vi "Binary (Approximate) Search 1D Array (DBL).vi"(1 "epsilon (machine)":dbl=2.220446049250313e-16, 2 "element":dbl format="%.2f", 3 "1D array":dbl[](array[numeric]) format="%.2f") -> (0 "index":i32)   [LabVIEW 2019]
doc: "This is a binary search through a 1D array. It has no start index input and searches the entire array for the element requested.\n\nIf found, the index of the match is returned. If not found, an index of -1 is returned.\n\nDue to the nature of the binary search, your input array must already be sorted. This function will not sort your array, so if you send in an unsorted array, it will not function properly. Furthermore, if you have duplicate elements in your array, it is not guaranteed that the index returned will be to the match with the lowest array element number.\n\nThis is the double-precision floating-point (DBL) portion of the polymorphic VI."
panel:
  # "Select Help»Show Context Help and move the cursor \nover the VI icon to display help for this VI."
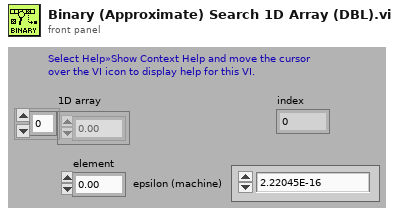
[diagram p1: front panel]
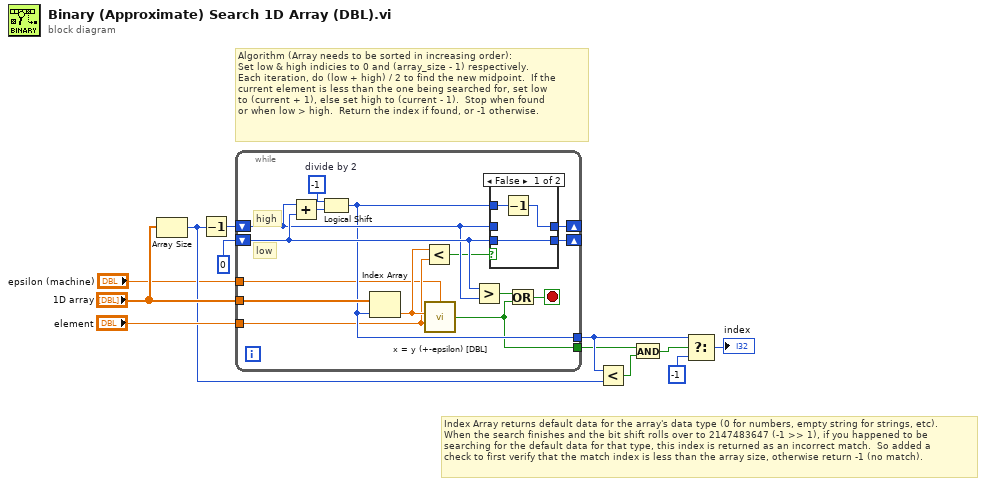
[diagram p0: block diagram]
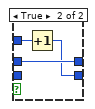
[diagram p2: hidden frame]
diagram:
  # "Index Array returns default data for the array's data type (0 for numbers, empty string for strings, etc).\nWhen the search finishes and the bit shift rolls over to 2147483647 (-1 >> 1), if you happened to be\nsearching for the default data for that type, this index is returned as an incorrect match.  So added a\ncheck to first verify that the match index is less than the array size, otherwise return -1 (no match)."
  # "Algorithm (Array needs to be sorted in increasing order):\nSet low & high indicies to 0 and (array_size - 1) respectively.\nEach iteration, do (low + high) / 2 to find the new midpoint.  If the\ncurrent element is less than the one being searched for, set low\nto (current + 1), else set high to (current - 1).  Stop when found\nor when low > high.  Return the index if found, or -1 otherwise."
  n1 = Array Size(array="1D array") -> (size(s)=w2:i32)
  n2 = Decrement(x=w2) -> (x-1=w9:i32)
  n3 = while {
    tunnel: "1D array" -> [w27]
    tunnel: "element" -> [w14]
    shift-right: [w23] -> _
    shift-left: w9 -> [w20]
    tunnel: [w16] -> w4
    shift-right: [w22] -> _
    shift-left: 0 -> [w21]
    tunnel: [w18] -> w5
    tunnel: "epsilon (machine)" -> [w13]
    stop <- w26 stop-if-true
    w24 = -1  # divide by 2
    # "low"
    # "high"
    n4 = Add(x=w20, y=w21) -> (x+y=w25:i32)
    n5 = Logical Shift(y=w24, x=w25) -> (x << y=w18:i32)
    n6 = Index Array(array=w27, index=w18) -> (element=w15:dbl)
    n7 = Less?(x=w15, y=w14) -> (x < y?=w19:bool)
    n8 = call "x = y (+-epsilon) [DBL].vi"("epsilon (machine)"=w13, "x"=w15, "y"=w14) -> ("x = y +/- epsilon"=w16:bool)  [unwired: 12 in]
    n9 = Greater?(x=w21, y=w20) -> (0:w17:bool)
    n10 = case shown="False" w19 {
      tunnel: w20 -> [_ w33]
      tunnel: w21 -> [w29 _]
      tunnel: [w28 w33] -> w23
      tunnel: w18 -> [w30 w32]
      tunnel: [w29 w31] -> w22
      frame False {
        n11 = Decrement(x=w30) -> (x-1=w28:i32)
      }
      frame True {
        n12 = Increment(x=w32) -> (x+1=w31:i32)
      }
    }
    n13 = Or(x=w17, y=w16) -> (x .or. y?=w26:bool)
  }
  n14 = Less?(x=w5, y=w2) -> (x < y?=w6:bool)
  n15 = And(x=w4, y=w6) -> (x .and. y?=w3:bool)
  n16 = Select(t=w5, s=w3, f=-1) -> (s? t:f=→"index":i32)
